vi "PAN_ShutdownActions.vi"(7 "cmdQ":refnum<queue>, 8 "shutdownscr ref":refnum<vi>) -> (2 "response":string)   [LabVIEW 2016]
uses:
  PAN_cmdStruct.ctl
panel:
  in  "element":T1
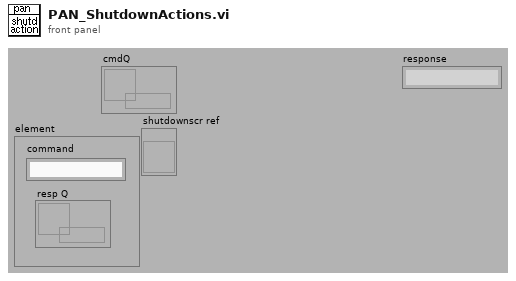
[diagram p1: front panel]
types:
  T1 = typedef "PAN_cmdStruct.ctl" = cluster{"command":string, "resp Q":refnum<queue>}
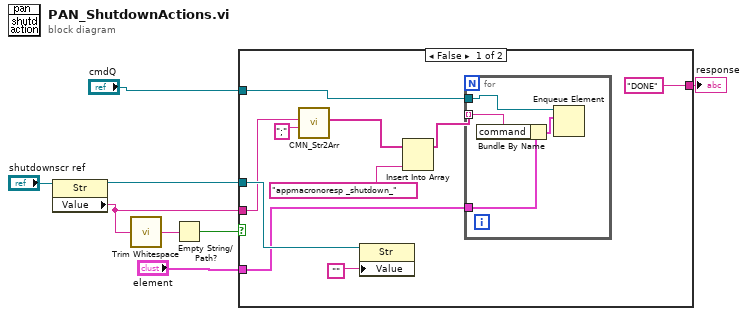
[diagram p0: block diagram]
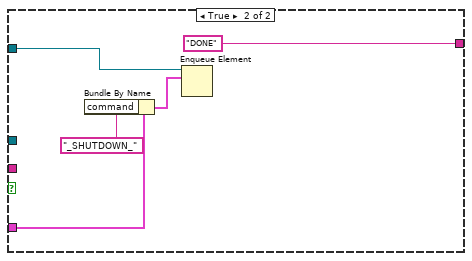
[diagram p2: hidden frame]
diagram:
  n1 = property class="Str"(reference="shutdownscr ref") -> (reference out=w6:refnum<vi>, "Value"=w1:string)  [unwired: 1 in, 1 out]
  n2 = call <vilib>:"Trim Whitespace.vi"("string"=w1) -> ("trimmed string"=w8:string)  [unwired: 1 in]
  n3 = Empty String/Path?(string/path=w8) -> (empty?=w7:bool)
  n4 = case shown="False" w7 {
    tunnel: w1 -> [w16 _]
    tunnel: "cmdQ" -> [w13 w27]
    tunnel: ["DONE" ("ImmedReplyString") "DONE" ("ImmedReplyString")] -> w2
    tunnel: w6 -> [w18 _]
    tunnel: "element" -> [w12 w25]
    frame False {
      n5 = call "CMN_Str2Arr.vi"("separator"=";", "string in"=w16) -> ("Array out"=w11:string[])  [unwired: 2 in, 7 out]
      n6 = property class="Str"(reference=w18, "Value"="") -> ()  [unwired: 1 in, 2 out]
      n7 = Insert Into Array(array=w11, new element="appmacronoresp _shutdown_" ("new element/subarray")) -> (w10:string[])  [unwired: 1 in]
      n8 = for {
        tunnel: w13 -> [w22]
        tunnel: w10 -> [w21] mode=indexing
        tunnel: w12 -> [w20]
        n9 = Bundle By Name(cluster=w20, "command"=w21) -> (w19:T1)
        n10 = Enqueue Element(queue=w22, element=w19) -> ()  [unwired: 1 in, 4 out]
      }
    }
    frame True {
      n11 = Bundle By Name(cluster=w25, "command"="_SHUTDOWN_") -> (w24:T1)
      n12 = Enqueue Element(queue=w27, element=w24) -> ()  [unwired: 1 in, 4 out]
    }
  }
  "response" <- w2
